vi "create_filename_iteration_string.vi"(8 "error in (no error)":errorcluster, 9 "variable indices":i32[](array[numeric]), 10 "Variable Names Array":string[](array[string])) -> (0 "error out":errorcluster, 3 "XYZ iteration string":string)   [LabVIEW 2011]
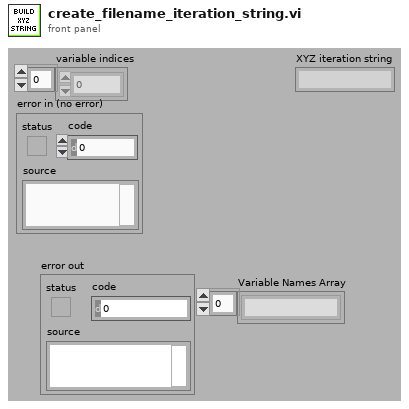
[diagram p1: front panel]
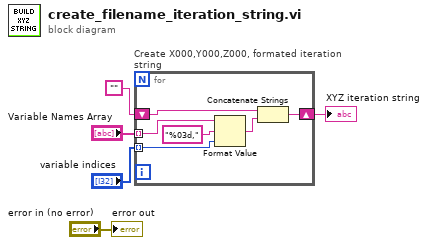
[diagram p0: block diagram]
diagram:
  n1 = for "Create X000,Y000,Z000, formated iteration string" {
    tunnel: "Variable Names Array" -> [w10] mode=indexing
    tunnel: "variable indices" -> [w11] mode=indexing
    shift-right: [w7] -> w1
    shift-left: "" -> [w6]
    n2 = Format Value(string ("")=w10, format string="%03d,", value (0)=w11) -> (output string=w8:string)
    n3 = Concatenate Strings(w6, w8) -> (w7:string)
  }
  "XYZ iteration string" <- w1
  "error out" <- "error in (no error)"
